vi "MapPath.vi"(9 "All Lines out":T1, 10 "ShowPath":T4[](array[typedef]), 11 "Array 2":cluster{cluster{"X":dbl, "Z":dbl}[]}[](array[cluster])) -> (3 "Array":cluster{cluster{"X":dbl, "Z":dbl}[]}[](array[cluster]))   [LabVIEW 2014]
uses:
  Components/PathFinder/Controls/PathControl.ctl
  Libraries/Map Data Folder/All-Lines.ctl
  Libraries/Map Data Folder/LineCluster.ctl
  Libraries/Map Data Folder/LineConnection.ctl
  Libraries/Map Data Folder/Map Data.lvlib
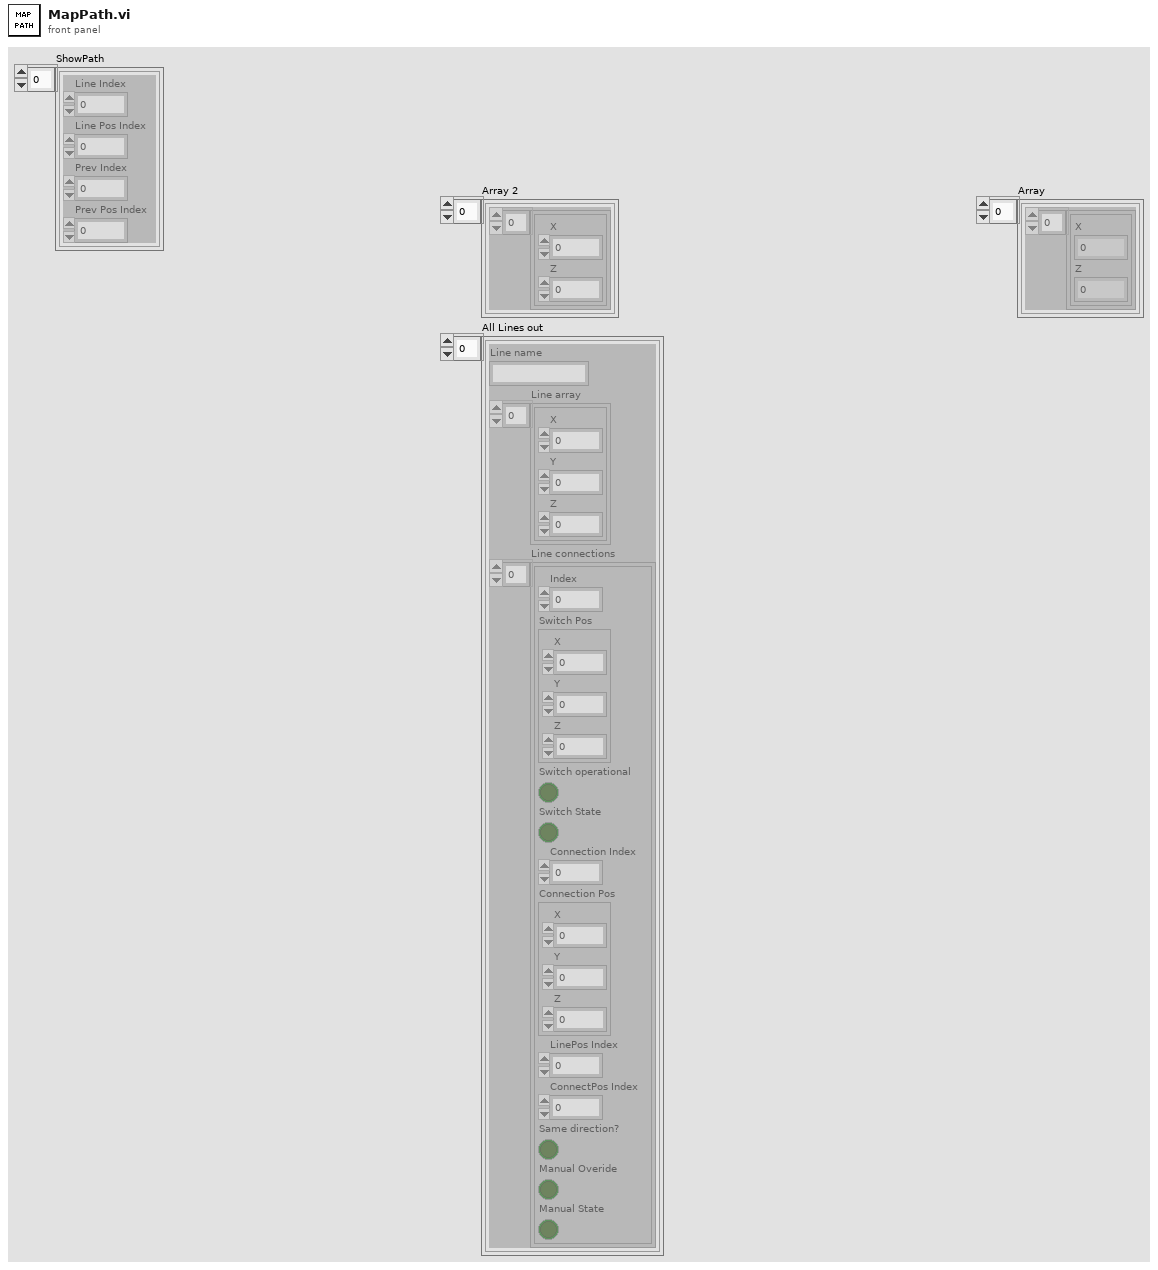
[diagram p1: front panel]
types:
  T1 = typedef "Map Data.lvlib/All-Lines.ctl" = T2[]
  T2 = typedef "Map Data.lvlib/LineCluster.ctl" = cluster{"Line name":string, "Line array":cluster{"X":dbl, "Y":dbl, "Z":dbl}[], "Line connections":T3[]}
  T3 = typedef "Map Data.lvlib/LineConnection.ctl" = cluster{"Index":i32, "Switch Pos":cluster{"X":dbl, "Y":dbl, "Z":dbl}, "Switch operational":bool, "Switch State":bool, "Connection Index":i32, "Connection Pos":cluster{"X":dbl, "Y":dbl, "Z":dbl}, "LinePos Index":i32, "ConnectPos Index":i32, "Same direction?":bool, "Manual Overide":bool, "Manual State":bool}
  T4 = typedef "PathControl.ctl" = cluster{"Line Index":i32, "Line Pos Index ":i32, "Prev Index ":i32, "Prev Pos Index":i32}
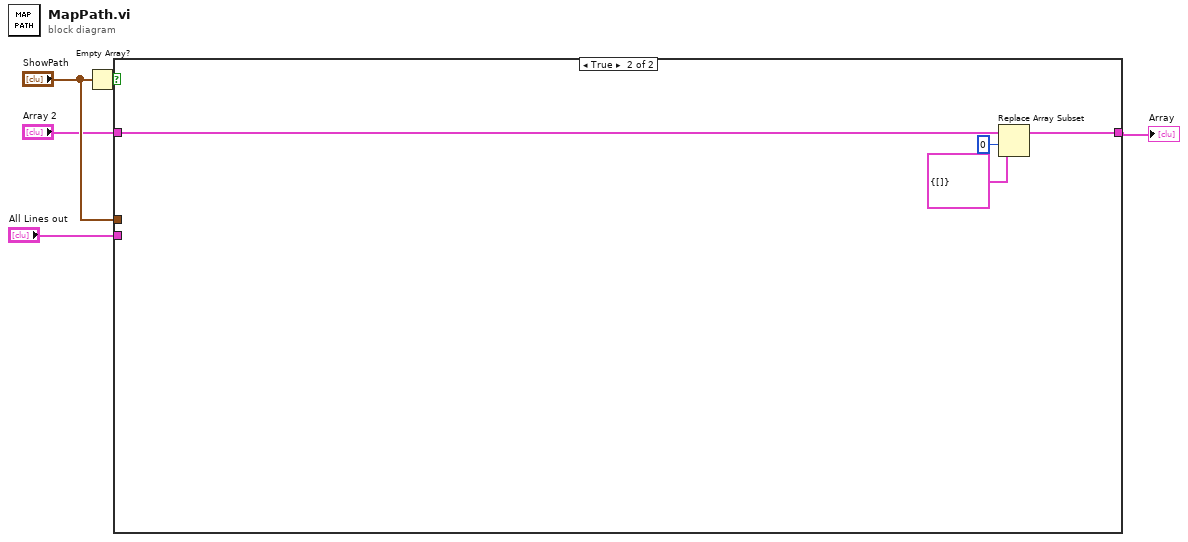
[diagram p0: block diagram]
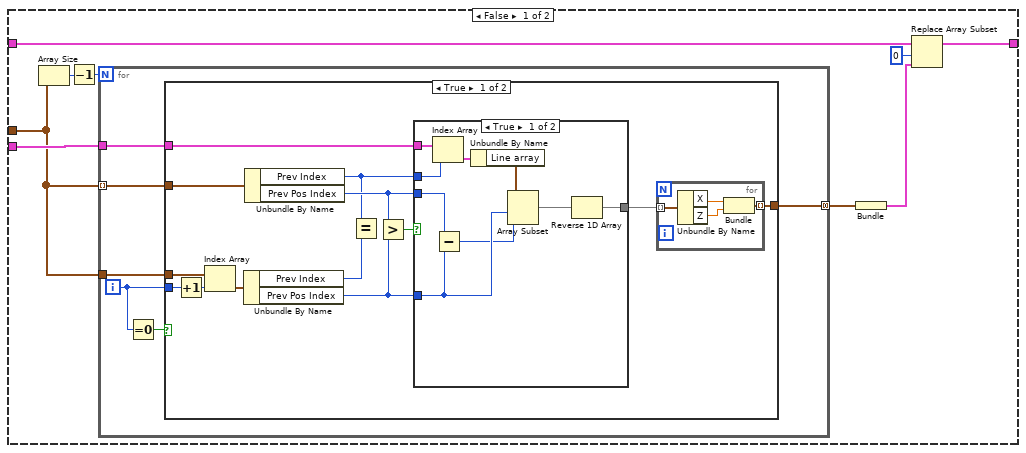
[diagram p2: hidden frame]
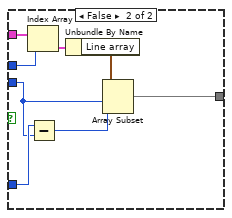
[diagram p3: hidden frame]
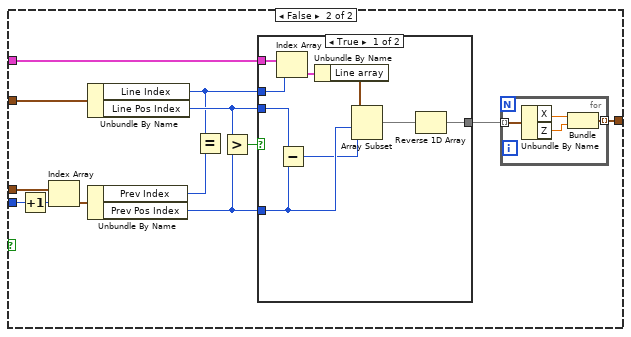
[diagram p4: hidden frame]
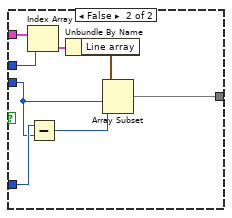
[diagram p5: hidden frame]
diagram:
  n1 = Empty Array?(array="ShowPath") -> (empty?=w5:bool)
  n2 = case shown="True" w5 {
    tunnel: "Array 2" -> [w12 w91]
    tunnel: [w11 w90] -> w2
    tunnel: "ShowPath" -> [w8 _]
    tunnel: "All Lines out" -> [w14 _]
    frame False {
      n3 = Array Size(array=w8) -> (size(s)=w7:i32)
      n4 = Decrement(x=w7) -> (x-1=w6:i32)
      n5 = for {
        N: w6 -> [_]
        tunnel: w8 -> [w20] mode=indexing
        tunnel: w8 -> [w19]
        tunnel: w14 -> [w18]
        tunnel: [w17] -> w13 mode=concatenating
        i -> [w16]
        n6 = Equal To 0?(x=w16) -> (x = 0?=w15:bool)
        n7 = case shown="True" w15 {
          tunnel: w20 -> [w33 w67]
          tunnel: w19 -> [w32 w66]
          tunnel: w16 -> [w31 w65]
          tunnel: w18 -> [w26 w60]
          tunnel: [w21 w55] -> w17
          frame True {
            n8 = Increment(x=w31) -> (x+1=w30:i32)
            n9 = Index Array(array=w32, index=w30) -> (element=w29:T4)
            n10 = Unbundle By Name(w29) -> ("Prev Index"=w28:i32, "Prev Pos Index"=w24:i32)
            n11 = Unbundle By Name(w33) -> ("Prev Index"=w23:i32, "Prev Pos Index"=w25:i32)
            n12 = Equal?(x=w23, y=w28) -> ()  [unwired: 1 out]
            n13 = Greater?(x=w25, y=w24) -> (0:w27:bool)
            n14 = case shown="True" w27 {
              tunnel: w26 -> [w45 w54]
              tunnel: w25 -> [w46 w47]
              tunnel: w24 -> [w41 w48]
              tunnel: w23 -> [w44 w53]
              tunnel: [w38 w49] -> w22
              frame True {
                n15 = Index Array(array=w45, index=w44) -> (element=w43:T2)
                n16 = Subtract(x=w46, y=w41) -> (x-y=w40:i32)
                n17 = Unbundle By Name(w43) -> ("Line array"=w42:cluster{"X":dbl, "Y":dbl, "Z":dbl}[])
                n18 = Array Subset(array=w42, index=w41, length=w40) -> (w39:cluster{"X":dbl, "Y":dbl, "Z":dbl}[])
                n19 = Reverse 1D Array(array=w39) -> (reversed array=w38:cluster{"X":dbl, "Y":dbl, "Z":dbl}[])
              }
              frame False {
                n20 = Index Array(array=w54, index=w53) -> (element=w52:T2)
                n21 = Subtract(x=w48, y=w47) -> (x-y=w50:i32)
                n22 = Unbundle By Name(w52) -> ("Line array"=w51:cluster{"X":dbl, "Y":dbl, "Z":dbl}[])
                n23 = Array Subset(array=w51, index=w47, length=w50) -> (w49:cluster{"X":dbl, "Y":dbl, "Z":dbl}[])
              }
            }
            n24 = for {
              tunnel: w22 -> [w37] mode=indexing
              tunnel: [w34] -> w21 mode=indexing
              n25 = Unbundle By Name(w37) -> ("X"=w36:dbl, "Z"=w35:dbl)
              n26 = Bundle("X"=w36, "Z"=w35) -> (w34:cluster{"X":dbl, "Z":dbl})  [unwired: 1 in]
            }
          }
          frame False {
            n27 = Increment(x=w65) -> (x+1=w64:i32)
            n28 = Index Array(array=w66, index=w64) -> (element=w63:T4)
            n29 = Unbundle By Name(w67) -> ("Line Index"=w57:i32, "Line Pos Index"=w59:i32)
            n30 = Unbundle By Name(w63) -> ("Prev Index"=w62:i32, "Prev Pos Index"=w58:i32)
            n31 = Equal?(x=w57, y=w62) -> ()  [unwired: 1 out]
            n32 = Greater?(x=w59, y=w58) -> (0:w61:bool)
            n33 = case shown="True" w61 {
              tunnel: w60 -> [w79 w88]
              tunnel: w59 -> [w80 w81]
              tunnel: w58 -> [w75 w82]
              tunnel: w57 -> [w78 w87]
              tunnel: [w72 w83] -> w56
              frame True {
                n34 = Index Array(array=w79, index=w78) -> (element=w77:T2)
                n35 = Subtract(x=w80, y=w75) -> (x-y=w74:i32)
                n36 = Unbundle By Name(w77) -> ("Line array"=w76:cluster{"X":dbl, "Y":dbl, "Z":dbl}[])
                n37 = Array Subset(array=w76, index=w75, length=w74) -> (w73:cluster{"X":dbl, "Y":dbl, "Z":dbl}[])
                n38 = Reverse 1D Array(array=w73) -> (reversed array=w72:cluster{"X":dbl, "Y":dbl, "Z":dbl}[])
              }
              frame False {
                n39 = Index Array(array=w88, index=w87) -> (element=w86:T2)
                n40 = Subtract(x=w82, y=w81) -> (x-y=w84:i32)
                n41 = Unbundle By Name(w86) -> ("Line array"=w85:cluster{"X":dbl, "Y":dbl, "Z":dbl}[])
                n42 = Array Subset(array=w85, index=w81, length=w84) -> (w83:cluster{"X":dbl, "Y":dbl, "Z":dbl}[])
              }
            }
            n43 = for {
              tunnel: w56 -> [w71] mode=indexing
              tunnel: [w68] -> w55 mode=indexing
              n44 = Unbundle By Name(w71) -> ("X"=w70:dbl, "Z"=w69:dbl)
              n45 = Bundle("X"=w70, "Z"=w69) -> (w68:cluster{"X":dbl, "Z":dbl})  [unwired: 1 in]
            }
          }
        }
      }
      n46 = Bundle(w13) -> (w10:cluster{cluster{"X":dbl, "Z":dbl}[]})  [unwired: 1 in]
      n47 = Replace Array Subset(array=w12, new element=w10, index=0) -> (w11:cluster{cluster{"X":dbl, "Z":dbl}[]}[])
    }
    frame True {
      n48 = Replace Array Subset(array=w91, new element=cluster{cluster{"X":dbl, "Z":dbl}[]} {[]} ("new element/subarray"), index=0) -> (w90:cluster{cluster{"X":dbl, "Z":dbl}[]}[])
    }
  }
  "Array" <- w2
